vi "Constructor.vi"(8 "error in (no error)":errorcluster, 11 "Marinara in":refnum<class "Marinara.lvclass">) -> (0 "error out":errorcluster, 2 "Ingredients":string, 3 "Marinara out":refnum<class "Marinara.lvclass">)   [LabVIEW 2013, in "Marinara.lvclass"]
uses:
  Marinara.lvclass
panel:
  # "§Ú¬O¤j»[Âæ"
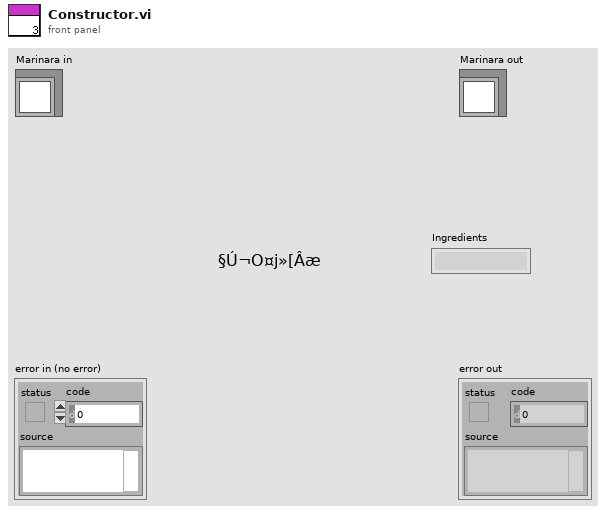
[diagram p1: front panel]
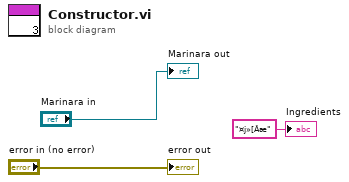
[diagram p0: block diagram]
diagram:
  "error out" <- "error in (no error)"
  "Marinara out" <- "Marinara in"
  "Ingredients" <- "¤j»[Âæ" ("Ingredients")
